vi "Launch Model.vi"(8 "error in (no error)":errorcluster, 11 "IViewModel In":refnum<class "IViewModel.lvclass">) -> (0 "error out":errorcluster, 3 "IViewModel Out":refnum<class "IViewModel.lvclass">)   [LabVIEW 2015, in "IViewModel.lvlib" / "IViewModel.lvclass"]
doc: "<License>\nCopyright © 2017 Composed Systems, LLC | All rights reserved\nwww.composed.io\n\nAuthor: Ethan Stern <ethan.stern@composed.io>\n\nThis software is provided \"AS IS\" WITHOUT WARRANTIES, either express or implied, AND IS FOR EDUCATIONAL PURPOSES ONLY.\n</License>"
uses:
  IViewModel.lvclass
  IMediator/IMediator Messages/Publish Msg/Publish Msg.lvclass
  IViewModel.lvclass/IViewModel.ctl
  AbstractMessages/PreAddressedMsg/PreAddressedMsg.lvclass/PreAddressedMsg.ctl
  IModel/IModel/IModel.lvclass/IModel.ctl
  <vilib>/ActorFramework/Actor/Actor.lvclass
  IModel/IModel/IModel.lvclass
  AbstractMessages/PreAddressedMsg/PreAddressedMsg.lvclass
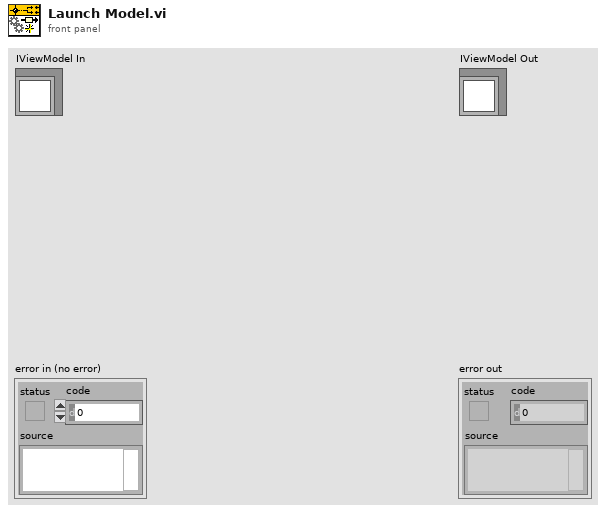
[diagram p1: front panel]
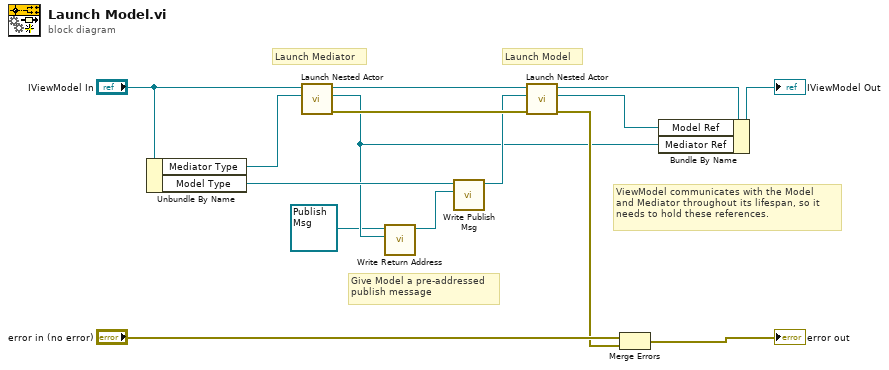
[diagram p0: block diagram]
diagram:
  # "Launch Model"
  # "Launch Mediator"
  # "Give Model a pre-addressed\npublish message"
  # "ViewModel communicates with the Model\nand Mediator throughout its lifespan, so it\nneeds to hold these references."
  n1 = Unbundle By Name("IViewModel In") -> ("Mediator Type"=w12:refnum<class "IMediator.lvclass">, "Model Type"=w11:refnum<class "IModel.lvclass">)
  n2 = call <vilib>:"Launch Nested Actor.vi"("Nested Actor"=w12, "Caller Actor in"="IViewModel In") -> ("error out"=w7:errorcluster, "Nested Actor's Enqueuer"=w3:refnum<class "Message Enqueuer.lvclass">, "Caller Actor out"=w13:refnum<class "IViewModel.lvclass">)  [unwired: 7 in]
  n3 = call "Write Return Address.vi"("Return Address"=w3, "PreAddressedMsg in"=refnum<class "Publish Msg.lvclass"> refnum ("IMediator.lvlib:Publish Msg.lvclass")) -> ("PreAddressedMsg out"=w2:refnum<class "Publish Msg.lvclass">)  [unwired: 9 in]
  n4 = call "Write Publish Msg.vi"("Pre-Addressed Publish Msg"=w2, "IModel in"=w11) -> ("IModel out"=w4:refnum<class "IModel.lvclass">)  [unwired: 9 in]
  n5 = call <vilib>:"Launch Nested Actor.vi"("error in (no error)"=w7, "Nested Actor"=w4, "Caller Actor in"=w13) -> ("error out"=w5:errorcluster, "Nested Actor's Enqueuer"=w8:refnum<class "Message Enqueuer.lvclass">, "Caller Actor out"=w10:refnum<class "IViewModel.lvclass">)  [unwired: 6 in]
  n6 = Merge Errors("error in (no error)", w5) -> (→"error out":errorcluster)
  n7 = Bundle By Name(cluster=w10, "Model Ref"=w8, "Mediator Ref"=w3) -> (→"IViewModel Out":refnum<class "IViewModel.lvclass">)
